vi "calculateDeltaTimestamp.vi"(8 "error in (no error)":errorcluster, 11 "ChirpWave in":refnum<class "ChirpWave.lvclass">) -> (0 "error out":errorcluster, 2 "Delta Timestamp":dbl format="%.9f", 3 "ChirpWave out":refnum<class "ChirpWave.lvclass">)   [LabVIEW 2015, in "ChirpWave.lvclass"]
uses:
  ChirpWave.lvclass
  ChirpWave.lvclass/ChirpWave.ctl
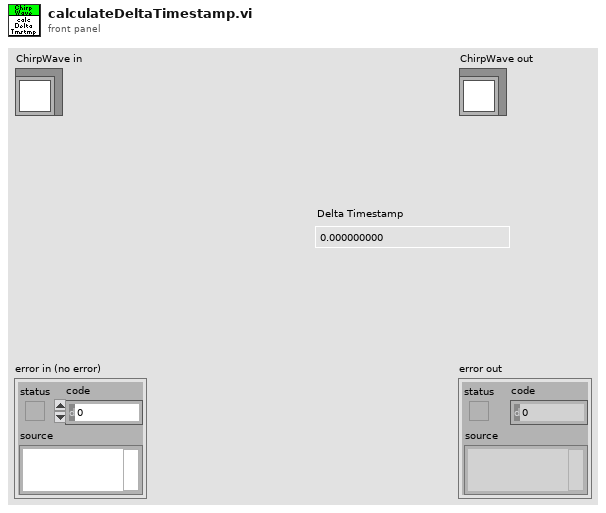
[diagram p1: front panel]
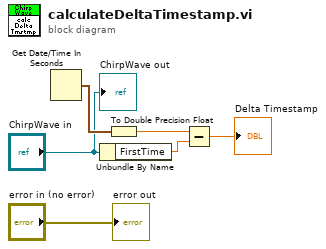
[diagram p0: block diagram]
diagram:
  n1 = Get Date/Time In Seconds() -> (seconds since 1Jan1904=w5:timestamp)
  n2 = Unbundle By Name("ChirpWave in") -> ("FirstTime"=w2:dbl)
  n3 = To Double Precision Float(number=w5) -> (double precision float=w3:dbl)
  n4 = Subtract(x=w3, y=w2) -> (x-y=→"Delta Timestamp":dbl)
  "error out" <- "error in (no error)"
  "ChirpWave out" <- "ChirpWave in"
